vi "bin2fixed30.vi"(9 "number":u32) -> (1 "Result":ext)   [LabVIEW 2020]
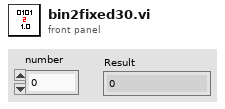
[diagram p1: front panel]
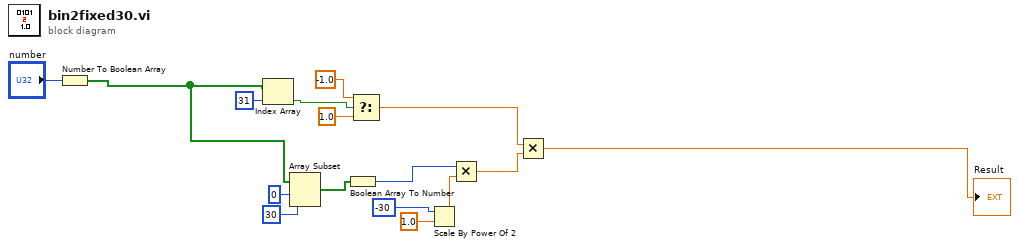
[diagram p0: block diagram]
diagram:
  n1 = Number To Boolean Array(number="number") -> (Boolean array=w2:bool[])
  n2 = Index Array(array=w2, index=31) -> (element=w4:bool)
  n3 = Array Subset(array=w2, index=0, length=30) -> (w3:bool[])
  n4 = Boolean Array To Number(Boolean array=w3) -> (number=w7:u32)
  n5 = Select(t=-1.0, s=w4, f=1.0) -> (s? t:f=w11:dbl)
  n6 = Scale By Power Of 2(n=i16 -30, x=1.0) -> (x*2^n=w8:dbl)
  n7 = Multiply(x=w7, y=w8) -> (x*y=w6:dbl)
  n8 = Multiply(x=w11, y=w6) -> (x*y=→"Result":dbl)
